vi "Step Execution Start.vi"(8 "error in (no error)":errorcluster, 11 "Execution in":refnum<data-value>) -> (0 "error out":errorcluster, 2 "Step":refnum<class "Step.lvclass">, 3 "Execution out":refnum<data-value>)   [LabVIEW 2015, in "Execution.lvclass"]
uses:
  Execution.lvclass
  Step.lvclass
  EXECUTION_UI_MSG.ctl
  Send UI Message.vi
  Project.lvclass
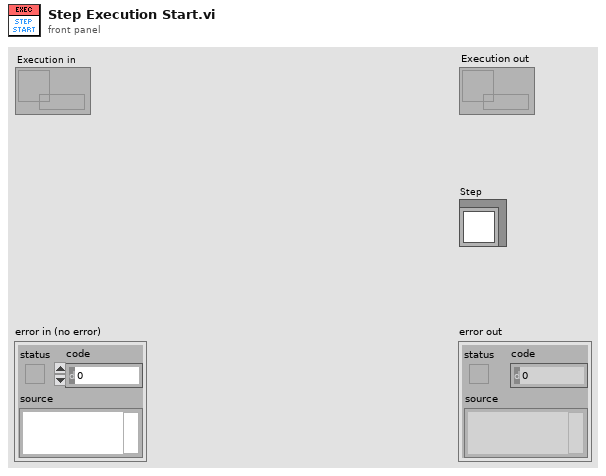
[diagram p1: front panel]
types:
  T1 = typedef "Execution.lvclass/EXECUTION_UI_MSG.ctl" = enum16{"EXECUTION_STATUS", "INIT_UI", "DUT_UPDATE", "BOTTOM_PANEL_UPDATE", "TOP_PANEL_UPDATE", "STEP_START", "STEP_END", "DISPLAY_RESULT", "APPLICATION_END"}
  T2 = typedef "Execution.lvclass/STEP_CONTEXT.ctl" = cluster{"StepIndex":u32, "Step":refnum<class "Step.lvclass">, "StartTime":timestamp, "EndTime":timestamp, "Result":T3, "Error Info":string, "Output Values":cluster{"Name":string, "Variant Data":variant}[]}
  T3 = typedef "Step.lvclass/STEP_STATUS.ctl" = enum16{"Skipped", "Done", "Passed", "Failed", "Error"}
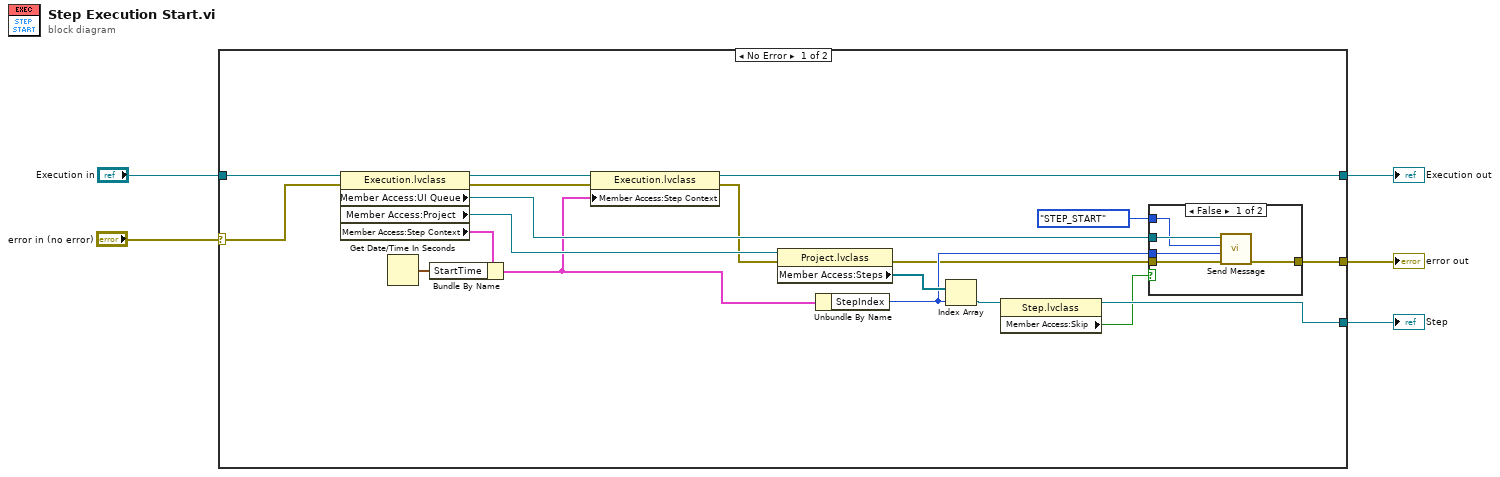
[diagram p0: block diagram]
diagram:
  n1 = case shown="No Error" "error in (no error)" {
    selector: "error in (no error)" -> [w23 w32]
    tunnel: [w14 w32] -> w4
    tunnel: [w6 w31] -> w1
    tunnel: "Execution in" -> [w7 w31]
    tunnel: [w20 _] -> w3
    frame No Error {
      n2 = property class="Execution.lvclass"(reference=w7, error in=w23) -> (reference out=w12:refnum<data-value>, error out=w11:errorcluster, "Member Access:UI Queue"=w18:refnum<queue>, "Member Access:Project"=w24:refnum<class "Project.lvclass">, "Member Access:Step Context"=w13:T2)
      n3 = Get Date/Time In Seconds() -> (seconds since 1Jan1904=w10:timestamp)
      n4 = Bundle By Name(cluster=w13, "StartTime"=w10) -> (w9:T2)
      n5 = property class="Execution.lvclass"(reference=w12, error in=w11, "Member Access:Step Context"=w9) -> (reference out=w6:refnum<data-value>, error out=w8:errorcluster)
      n6 = property class="Project.lvclass"(reference=w24, error in=w8) -> (error out=w16:errorcluster, "Member Access:Steps"=w22:refnum<class "Step.lvclass">[])  [unwired: 1 out]
      n7 = Unbundle By Name(w9) -> ("StepIndex"=w17:u32)
      n8 = Index Array(array=w22, index=w17) -> (element=w21:refnum<class "Step.lvclass">)
      n9 = property class="Step.lvclass"(reference=w21) -> (reference out=w20:refnum<class "Step.lvclass">, "Member Access:Skip"=w19:bool)  [unwired: 1 in, 1 out]
      n10 = case shown="False" w19 {
        tunnel: w18 -> [w29 _]
        tunnel: w17 -> [w28 _]
        tunnel: w16 -> [w27 w30]
        tunnel: EXECUTION_UI_MSG."STEP_START" ("Msg") -> [w26 _]
        tunnel: [w25 w30] -> w14
        frame False {
          n11 = call-poly "Send Message.vi"("error in (no error)"=w27, "Data"=w28, "Msg"=w26, "UI Queue"=w29) -> ("error out"=w25:errorcluster)  [unwired: 7 in]
        }
        frame True {
        }
      }
    }
    frame Error {
    }
  }
  "error out" <- w4
  "Step" <- w3
  "Execution out" <- w1
